vi "Asylum_SetOutWavePair.vi"(5 "whichBank":i32, 6 "interpolation":i32, 7 "eventString":string, 8 "error in (no error)":errorcluster, 9 "Wave B":cluster{"channelStringB":string, "waveB":string}, 10 "Wave A":cluster{"channelStringA":string, "waveA":string}, 11 "Application":refnum<k7>) -> (0 "error out":errorcluster, 3 "Application":refnum<k7>)   [LabVIEW 2016]
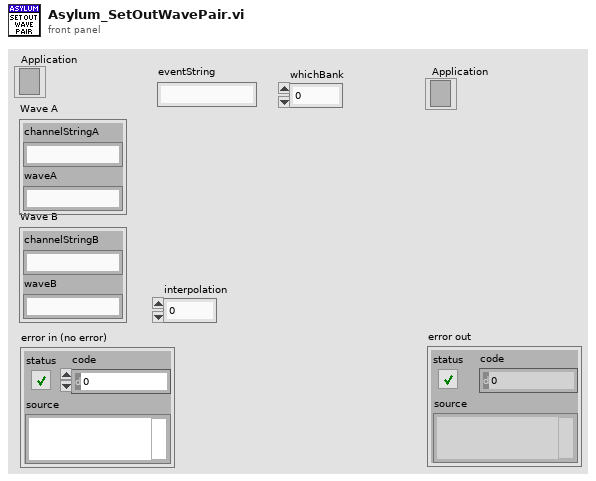
[diagram p1: front panel]
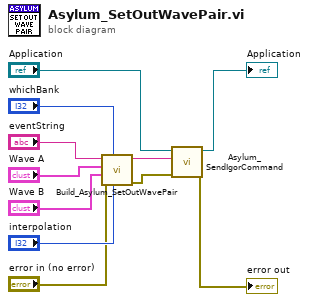
[diagram p0: block diagram]
diagram:
  n1 = call "Build_Asylum_SetOutWavePair.vi"("interpolation"="interpolation", "whichBank"="whichBank", "error in (no error)"="error in (no error)", "Wave B"="Wave B", "Wave A"="Wave A", "eventString"="eventString") -> ("error out"=w3:errorcluster, "Command"=w5:string)  [unwired: 4 in]
  n2 = call "Asylum_SendIgorCommand.vi"("error in (no error)"=w3, "command"=w5, "Application"="Application") -> ("error out"=→"error out":errorcluster, "Application"=→"Application":refnum<k7>)  [unwired: 5 in, 2 out]
